vi "Camera Receiver Loop.vi"() -> ()   [LabVIEW 2009]
uses:
  <vilib>/Platform/TimedLoop/XDataNode/XDataNode.xnode
  <vilib>/Platform/TimedLoop/XDataNode/loadlvalarms.vi
  <vilib>/Platform/TimedLoop/XDataNode/timing_clust.ctl
  <vilib>/Platform/TimedLoop/XDataNode/nitl_modes.ctl
  <vilib>/Platform/TimedLoop/XDataNode/wakeup.ctl
  Functional Global Variables/Actions for FG's.ctl
  TypeDefs/Sensor TypeDefs/SICK Array.ctl
  UI Comm/Watchdog Dish Labels.ctl
  <vilib>/Platform/TimedLoop/XDataNode/XDNodeRunTimeDep.lvlib
panel:
  out "Camera SICK":u16[](graph)
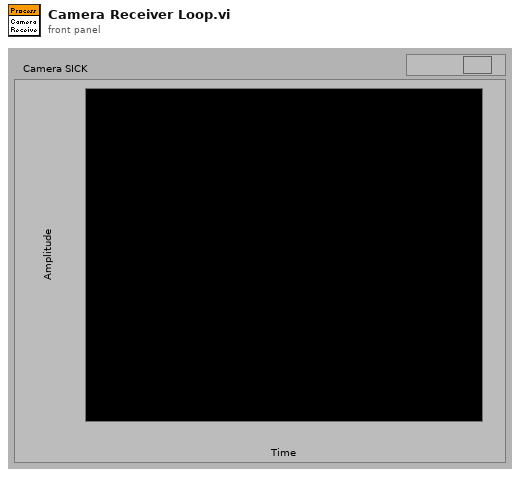
[diagram p1: front panel]
types:
  T1 = typedef "XDNodeRunTimeDep.lvlib/timing_clust.ctl" = cluster{"Expected End [f-1]":u64, "Actual End [f-1]":u64, "Finished Late? [f-1]":bool, "Expected End [i-1]":u64, "Actual End [i-1]":u64, "Finished Late? [i-1]":bool, "Expected Start [i]":u64, "Actual Start [i]":u64, "Expected Start [f]":u64, "Actual Start [f]":u64, "Source Name":string, "Structure Name":string, "Period":i64, "Deadline":i64, "Offset":i64, "Start":i64, "Priority":i32, "Timeout":i32, "Mode":T2, "Wakeup Reason":T3, "Error":errorcluster, "Source Type":string, "Secondary Source Type":string, "Global End Time":u64, "Global Start Time":u64, "Frame Duration":u64, "Iteration Duration":u64, "Assigned CPU":i32, "I/O Scan Engine Mode":u32}
  T2 = typedef "XDNodeRunTimeDep.lvlib/nitl_modes.ctl" = enum32{"No Change", "Process missed periods, maintain original phase", "Discard missed periods, maintain original phase", "Process missed periods, ignore original phase", "Discard missed periods, ignore original phase"}
  T3 = typedef "XDNodeRunTimeDep.lvlib/wakeup.ctl" = enum32{"Normal", "Aborted", "Asynchronous wakeup", "Timing source error", "Timed loop error", "Timeout"}
  T4 = typedef "UDP Base.ctl" = cluster{"UDP Session":refnum<k16>, "UDP Socket Params":T5}
  T5 = typedef "UDP Socket Params.ctl" = cluster{"Local Port":u16, "Read Timeout":i32, "Write Timeout":i32}
  T6 = typedef "Actions for FG's.ctl" = enum16{"Read", "Write"}
  T7 = cluster{"Sick array":u16[], "Camera init":bool, "Objects Array":cluster{"X Coord":dbl[], "Y Coord":dbl[]}[], "EVS HB":bool}
  T8 = typedef "SICK Array.ctl" = u16[]
  T9 = typedef "Watchdog Dish Labels.ctl" = enum16{"GPS", "SICK", "Compass", "Cameras", "Motor Controller", "Debug", "RC Receiver"}
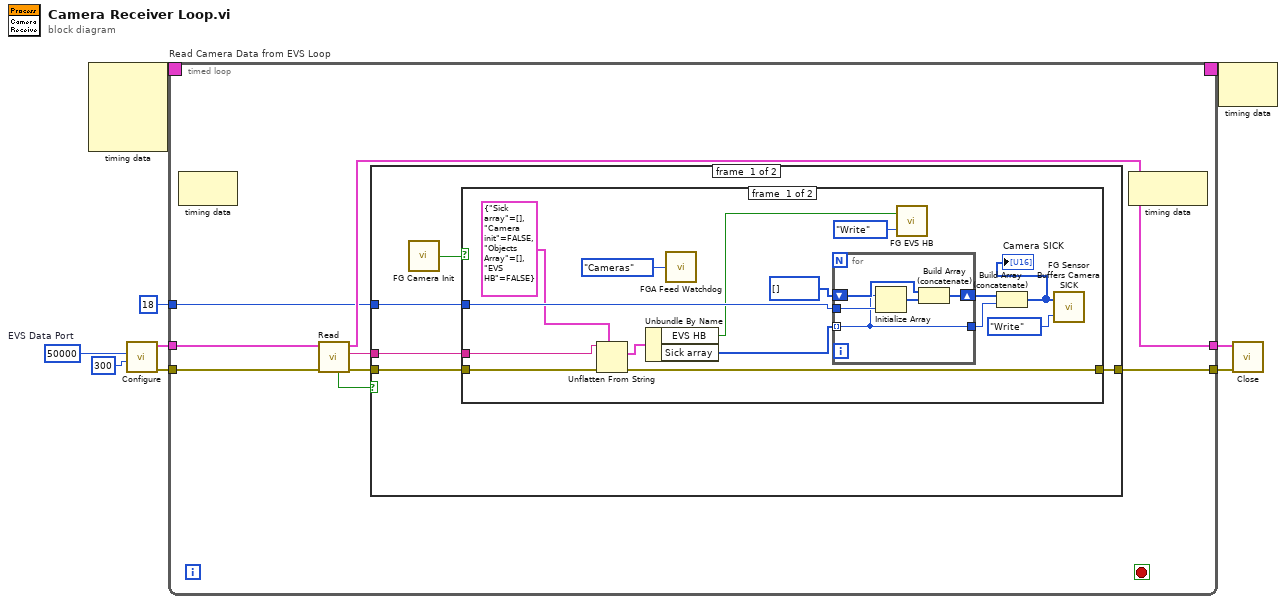
[diagram p0: block diagram]
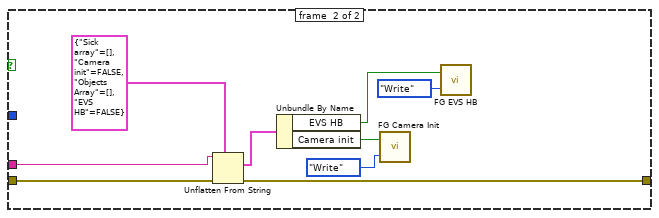
[diagram p2: hidden frame]
diagram:
  w6 = u16 50000  # EVS Data Port
  n1 = node-c288() -> (w2:T1)  [unwired: 4 in]
  n2 = call "Configure.vi"("Read Timeout"=300, "Local Port"=w6) -> ("error out"=w5:errorcluster, "UDP Base out"=w4:T4)  [unwired: 8 in]
  n3 = timed-loop "Read Camera Data from EVS Loop" {
    tunnel: w4 -> [w17]
    tunnel: w5 -> [w16]
    tunnel: [w13] -> w9
    tunnel: [w15] -> w8
    tunnel: 18 ("Numeric") -> [w14]
    timing: w2 -> [_]
    timing-out: [_] -> w1
    stop <- _ stop-if-true
    n4 = node-c288() -> ()  [unwired: 1 in, 1 out]
    n5 = call "Read.vi"("error in (no error)"=w16, "UDP Base in"=w17) -> ("error out"=w12:errorcluster, "Receive Data"=w11:string, "UDP Base out"=w15:T4, "Timeout"=w10:bool)  [unwired: 4 in, 2 out]
    n6 = case shown="False" w10 {
      tunnel: w12 -> [w22 w52]
      tunnel: [w21 w52] -> w13
      tunnel: w11 -> [w20 _]
      tunnel: w14 -> [w19 _]
      frame #0 {
        n7 = call "FG Camera Init.vi"() -> ("Camera Init out"=w18:bool)  [unwired: 2 in]
        n8 = case shown="True" w18 {
          tunnel: w22 -> [w37 w51]
          tunnel: [w34 w50] -> w21
          tunnel: w20 -> [w36 w49]
          tunnel: w19 -> [w32 _]
          frame #0 {
            n9 = Unflatten From String(type=T7 {"Sick array"=[], "Camera init"=FALSE, "Objects Array"=[], "EVS HB"=FALSE} ("output cluster"), binary string=w36, error in (no error)=w37) -> (value=w26:T7, error out=w34:errorcluster)  [unwired: 2 in, 1 out]
            n10 = Unbundle By Name(w26) -> ("EVS HB"=w23:bool, "Sick array"=w25:u16[])
            n11 = call "FGA Feed Watchdog.vi"("Watchdog Dish"=Watchdog_Dish_Labels."Cameras") -> ()  [unwired: 1 out]
            n12 = for {
              tunnel: w25 -> [w38] mode=indexing
              shift-right: [w40] -> w30
              shift-left: T8 [] ("SICK Data") -> [w42]
              tunnel: w32 -> [w39]
              tunnel: [w38] -> w29
              n13 = Initialize Array(w38, w39) -> (w41:u16[])
              n14 = Build Array (concatenate)(w42, w41) -> (w40:T8)
            }
            n15 = call "FG EVS HB.vi"("FG Action"=Actions_for_FG's."Write", "EVS HB In"=w23) -> ()  [unwired: 1 out]
            n16 = Build Array (concatenate)(w30, w29) -> (w28:T8)
            "Camera SICK" <- w28
            n17 = call "FG Sensor Buffers Camera SICK.vi"("FG Action (Read)"=Actions_for_FG's."Write", "Camera SICK Buffer in"=w28) -> ()  [unwired: 1 in, 1 out]
          }
          frame #1 {
            n18 = Unflatten From String(type=T7 {"Sick array"=[], "Camera init"=FALSE, "Objects Array"=[], "EVS HB"=FALSE} ("output cluster"), binary string=w49, error in (no error)=w51) -> (value=w48:T7, error out=w50:errorcluster)  [unwired: 2 in, 1 out]
            n19 = Unbundle By Name(w48) -> ("EVS HB"=w43:bool, "Camera init"=w47:bool)
            n20 = call "FG Camera Init.vi"("FG Action"=Actions_for_FG's."Write" ("FG Action (Read)"), "Camera Init in"=w47) -> ()  [unwired: 1 out]
            n21 = call "FG EVS HB.vi"("FG Action"=Actions_for_FG's."Write", "EVS HB In"=w43) -> ()  [unwired: 1 out]
          }
        }
      }
      frame #1 {
      }
    }
    n22 = node-c288() -> ()  [unwired: 1 in, 1 out]
  }
  n23 = node-c288(w1) -> ()  [unwired: 1 out]
  n24 = call "Close.vi"("error in (no error)"=w9, "Cluster of class private data"=w8) -> ()  [unwired: 9 in, 1 out]
